vi "Calculate Initial Rate.vi"(8 "error in (no error)":errorcluster, 10 "Position Change":i16, 11 "ScrollingList in":refnum<class "ScrollingList.lvclass">) -> (0 "error out":errorcluster, 3 "ScrollingList (dup)":refnum<class "ScrollingList.lvclass">)   [LabVIEW 2020, in "ScrollingList.lvclass"]
uses:
  ScrollingList.lvclass
  ScrollingList.lvclass/ScrollingList.ctl
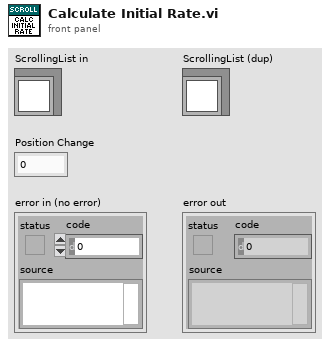
[diagram p1: front panel]
types:
  T1 = typedef "ScrollingList.lvclass/State Data.ctl" = cluster{"Timeout":i32, "Time":timestamp, "Y":i32, "Origin:Top":i16, "Rate":dbl, "ListItems":string[], "Item Height":i32, "Max Height":i32}
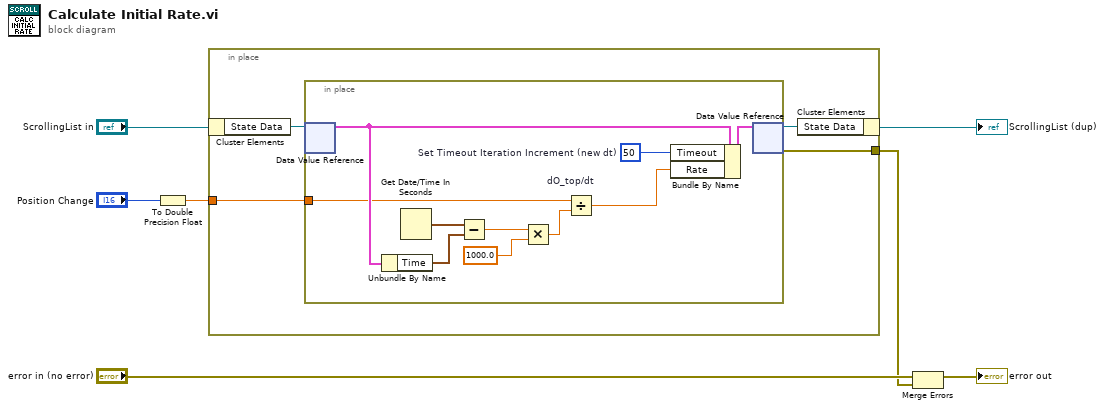
[diagram p0: block diagram]
diagram:
  n1 = To Double Precision Float(number="Position Change") -> (double precision float=w4:dbl)
  n2 = in-place {
    in-place-border: w4 -> [w9]
    in-place-border: [w8] -> w1
    n3 = in-place-cluster #1("ScrollingList in") -> ("State Data"=w11:refnum<data-value>)
    n4 = in-place {
      in-place-border: w9 -> [w15]
      w12 = 50  # Set Timeout Iteration Increment (new dt)
      n5 = in-place-dvr #2(w11) -> (w21:T1)  [unwired: 1 out]
      n6 = Unbundle By Name(w21) -> ("Time"=w18:timestamp)
      n7 = Get Date/Time In Seconds() -> (seconds since 1Jan1904=w19:timestamp)
      n8 = Subtract(x=w19, y=w18) -> (x-y=w16:dbl)
      n9 = Multiply(x=w16, y=1000.0) -> (x*y=w14:dbl)
      n10 = Divide "dO_top/dt"(x=w15, y=w14) -> (x/y=w13:dbl)
      n11 = Bundle By Name(cluster=w21, "Timeout"=w12, "Rate"=w13) -> (w20:T1)
      n12 = in-place-dvr #2(w20) -> (w10:refnum<data-value>, w8:errorcluster)
    }
    n13 = in-place-cluster #1("State Data"=w10) -> (→"ScrollingList (dup)":refnum<class "ScrollingList.lvclass">)
  }
  n14 = Merge Errors("error in (no error)", w1) -> (→"error out":errorcluster)
